vi "子VI-计算时间.vi"(11 "计算时间":i32) -> (3 "计算时间 2":i32)   [LabVIEW 2018]
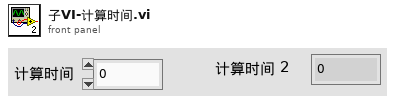
[diagram p1: front panel]
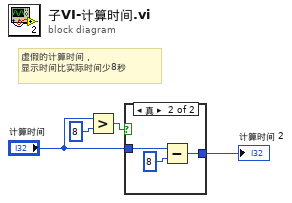
[diagram p0: block diagram]
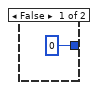
[diagram p2: hidden frame]
diagram:
  # "虚假的计算时间，\n显示时间比实际时间少8秒"
  n1 = Greater?(x="计算时间", y=8) -> (0:w3:bool)
  n2 = case shown="真" w3 {
    tunnel: "计算时间" -> [_ w8]
    tunnel: [0 w6] -> w1
    frame False {
    }
    frame True {
      n3 = Subtract(x=w8, y=8) -> (x-y=w6:i32)
    }
  }
  "计算时间 2" <- w1
